vi "GVSDataView Docking Process.vi"(8 "DataView Index":i32, 9 "Start Pos":T1, 11 "Mouse Pos":T1) -> (3 "StartPositin Out":T1)   [LabVIEW 2013]
uses:
  GVSNew View Global.vi
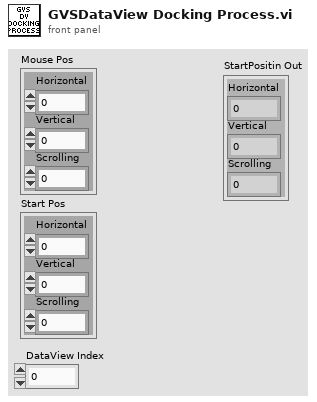
[diagram p1: front panel]
types:
  T1 = cluster{"Horizontal":i32, "Vertical":i32, "Scrolling":i32}
  T2 = typedef "Graph Main Info Cluster.ctl" = cluster{"Selected_BarIdx":i32, "Selected_PanelIdx":i32, "Graph Main VIRef":refnum<vi>, "ToolBarClick":bool, "Spliter Ref Array":refnum<vi>[], "Panel Ref Array":refnum<vi>[], "Spliter_matrix":i32[][], "Panel_matrix":i32[][], "child_spliterIdx_matrix":i32[][], "split_pos_matrix":i32[][], "Title State":bool, "sQueueName":string, "Frame nID":i32, "Graph VIRef Array":cluster{"Graph VIRef":refnum<vi>, "Panel Idx":i32, "Frame VIRef":refnum<vi>, "Icon Ring":i32, "Graph Type":string}[], "View Type":string}
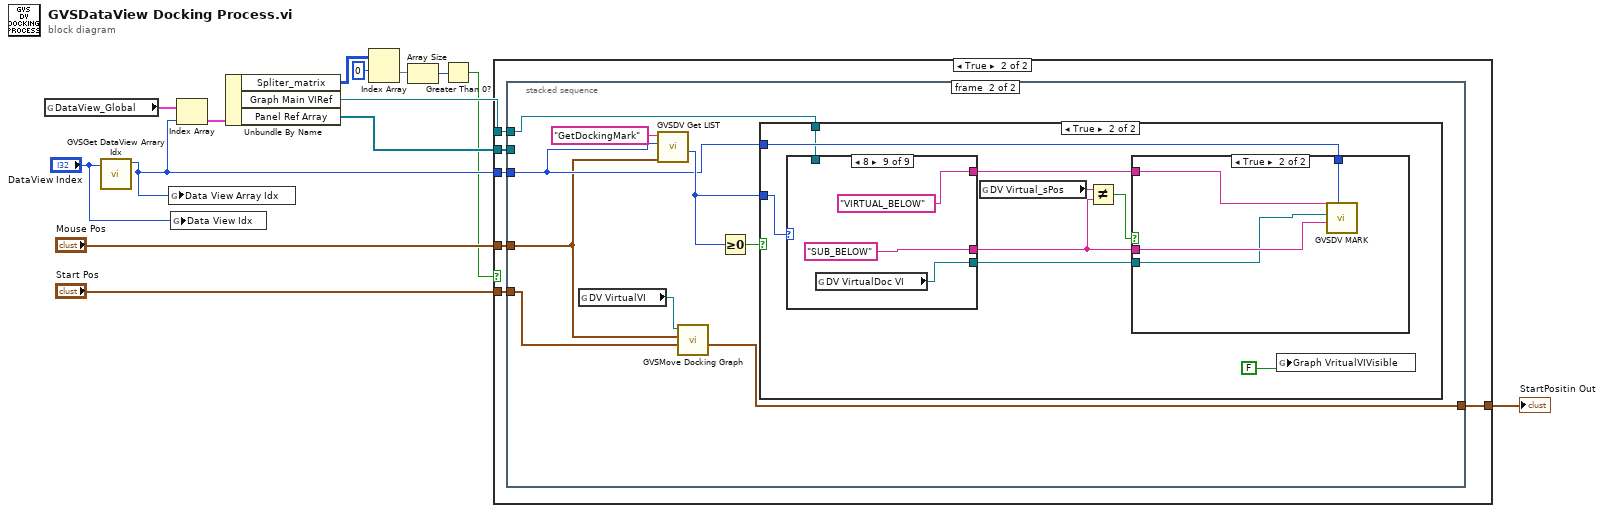
[diagram p0: block diagram]
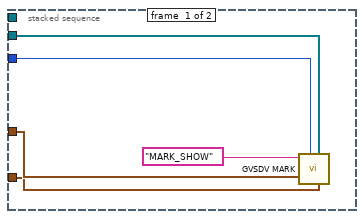
[diagram p3: hidden frame]
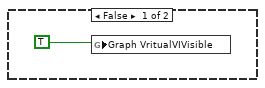
[diagram p4: hidden frame]
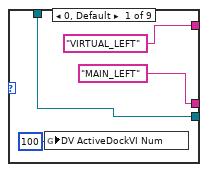
[diagram p6: hidden frame]
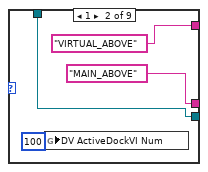
[diagram p7: hidden frame]
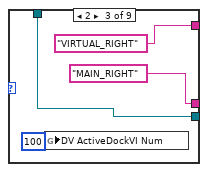
[diagram p8: hidden frame]
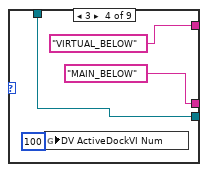
[diagram p9: hidden frame]
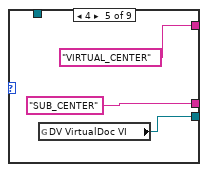
[diagram p10: hidden frame]
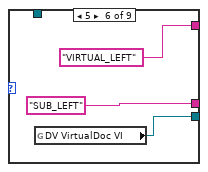
[diagram p11: hidden frame]
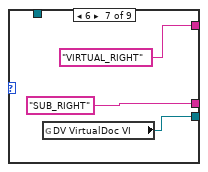
[diagram p12: hidden frame]
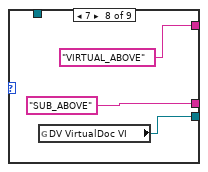
[diagram p13: hidden frame]
diagram:
  n1 = global read "GVSNew View Global.vi" "DataView_Global"() -> (w13:T2[])
  n2 = call "GVSGet DataView Arrary Idx.vi"("DataView Idx In"="DataView Index") -> ("DataView Arrary Idx out"=w3:i32)  [unwired: 10 in]
  n3 = global write "GVSNew View Global.vi" "Data View Array Idx"(w3) -> ()
  n4 = global write "GVSNew View Global.vi" "Data View Idx"("DataView Index") -> ()
  n5 = Index Array(array=w13, index=w3) -> (element=w12:T2)
  n6 = Unbundle By Name(w12) -> ("Spliter_matrix"=w9:i32[][], "Graph Main VIRef"=w10:refnum<vi>, "Panel Ref Array"=w11:refnum<vi>[])
  n7 = Index Array(array=w9, index (row)=0) -> (element=w7:i32[])  [unwired: 1 in]
  n8 = Array Size(array=w7) -> (size(s)=w6:i32)
  n9 = Greater Than 0?(x=w6) -> (x > 0?=w1:bool)
  n10 = case shown="True" w1 {
    tunnel: "Mouse Pos" -> [_ w21]
    tunnel: w3 -> [_ w20]
    tunnel: w11 -> [_ w19]
    tunnel: w10 -> [_ w18]
    tunnel: "Start Pos" -> [w15 w17]
    tunnel: [w15 w16] -> w5
    frame False {
    }
    frame True {
      n11 = stacked-sequence {
        tunnel: w21 -> [w23 w30]
        tunnel: w20 -> [w25 w31]
        tunnel: w19 -> [w24 _]
        tunnel: w18 -> [_ w32]
        tunnel: w17 -> [w22 w29]
        tunnel: [_ w27] -> w16
        frame #0 {
          n12 = call "GVSDV MARK.vi"("sAction"="MARK_SHOW", "MousePos"=w23, "DataView Array Index"=w25, "SubPanel array"=w24, "Start Pos In"=w22) -> ()  [unwired: 5 in, 1 out]
        }
        frame #1 {
          n13 = global read "GVSNew View Global.vi" "DV VirtualVI"() -> (w28:refnum<vi>)
          n14 = call "GVSDV Get LIST.vi"("sAction"="GetDockingMark", "DataView Array Index"=w31, "MousePos"=w30) -> ("nData_Out"=w33:i32)  [unwired: 4 in, 3 out]
          n15 = call "GVSMove Docking Graph.vi"("StartPositin In"=w29, "MousePositin In"=w30, "VI Ref In"=w28) -> ("StartPositin Out"=w27:T1)  [unwired: 6 in, 2 out]
          n16 = Greater Or Equal To 0?(x=w33) -> (x >= 0?=w34:bool)
          n17 = case shown="True" w34 {
            tunnel: w33 -> [_ w45]
            tunnel: w31 -> [_ w44]
            tunnel: w32 -> [_ w43]
            frame False {
              n18 = global write "GVSNew View Global.vi" "Graph VritualVIVisible"(TRUE ("VritualVIVisible")) -> ()
            }
            frame True {
              n19 = case shown="8" w45 {
                tunnel: ["MAIN_LEFT" ("sAction") "MAIN_ABOVE" ("sAction") "MAIN_RIGHT" ("sAction") "MAIN_BELOW" ("sAction") "SUB_CENTER" "SUB_LEFT" "SUB_RIGHT" "SUB_ABOVE" "SUB_BELOW"] -> w39
                tunnel: ["VIRTUAL_LEFT" ("sAction") "VIRTUAL_ABOVE" ("sAction") "VIRTUAL_RIGHT" ("sAction") "VIRTUAL_BELOW" ("sAction") "VIRTUAL_CENTER" "VIRTUAL_LEFT" "VIRTUAL_RIGHT" "VIRTUAL_ABOVE" "VIRTUAL_BELOW"] -> w40
                tunnel: w43 -> [w50 w54 w58 w62 _ _ _ _ _]
                tunnel: [w50 w54 w58 w62 w66 w69 w72 w75 w78] -> w37
                frame 0, Default {
                  n20 = global write "GVSNew View Global.vi" "DV ActiveDockVI Num"(100 ("ActiveDockVI Num")) -> ()
                }
                frame 1 {
                  n21 = global write "GVSNew View Global.vi" "DV ActiveDockVI Num"(100 ("ActiveDockVI Num")) -> ()
                }
                frame 2 {
                  n22 = global write "GVSNew View Global.vi" "DV ActiveDockVI Num"(100 ("ActiveDockVI Num")) -> ()
                }
                frame 3 {
                  n23 = global write "GVSNew View Global.vi" "DV ActiveDockVI Num"(100 ("ActiveDockVI Num")) -> ()
                }
                frame 4 {
                  n24 = global read "GVSNew View Global.vi" "DV VirtualDoc VI"() -> (w66:refnum<vi>)
                }
                frame 5 {
                  n25 = global read "GVSNew View Global.vi" "DV VirtualDoc VI"() -> (w69:refnum<vi>)
                }
                frame 6 {
                  n26 = global read "GVSNew View Global.vi" "DV VirtualDoc VI"() -> (w72:refnum<vi>)
                }
                frame 7 {
                  n27 = global read "GVSNew View Global.vi" "DV VirtualDoc VI"() -> (w75:refnum<vi>)
                }
                frame 8 {
                  n28 = global read "GVSNew View Global.vi" "DV VirtualDoc VI"() -> (w78:refnum<vi>)
                }
              }
              n29 = global read "GVSNew View Global.vi" "DV Virtual_sPos"() -> (w42:string)
              n30 = Not Equal?(x=w42, y=w39) -> (x != y?=w41:bool)
              n31 = case shown="True" w41 {
                tunnel: w40 -> [_ w49]
                tunnel: w39 -> [_ w48]
                tunnel: w44 -> [_ w47]
                tunnel: w37 -> [_ w46]
                frame False {
                }
                frame True {
                  n32 = call "GVSDV MARK.vi"("sAction"=w49, "mVritual_VIRef"=w46, "sData"=w48, "DataView Array Index"=w47) -> ()  [unwired: 6 in, 1 out]
                }
              }
              n33 = global write "GVSNew View Global.vi" "Graph VritualVIVisible"(FALSE ("VritualVIVisible")) -> ()
            }
          }
        }
      }
    }
  }
  "StartPositin Out" <- w5
